vi "ProducerConsumerDataVoorbeeld.vi"() -> ()   [LabVIEW 2019]
doc: "Use this template to build a producer/consumer design pattern. Use this template when you need to execute a process, such as data analysis, when a data source, such as a triggered acquisition, produces data at an uneven rate and you need to execute the process when the data becomes available."
panel:
  in  "stop":bool
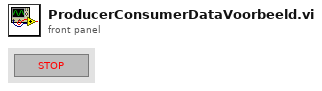
[diagram p1: front panel]
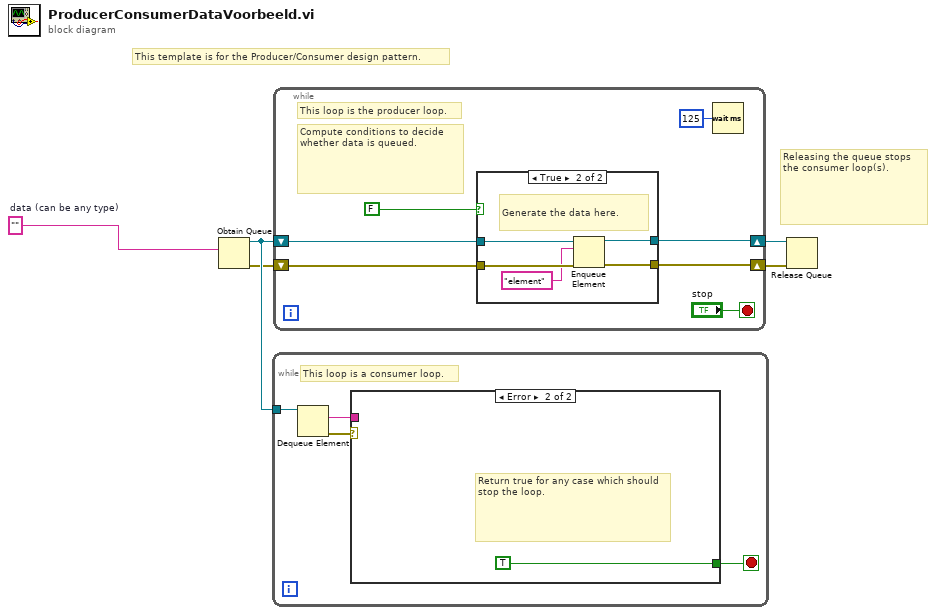
[diagram p0: block diagram]
diagram:
  w1 = ""  # data (can be any type)
  # "Releasing the queue stops the consumer loop(s)."
  # "This template is for the Producer/Consumer design pattern."
  n1 = Obtain Queue(element data type=w1) -> (queue out=w5:refnum<queue>, error out=w4:errorcluster)  [unwired: 4 in, 1 out]
  n2 = while {
    tunnel: w5 -> [w9]
    stop <- w6 stop-if-true
    # "This loop is a consumer loop."
    n3 = Dequeue Element(queue=w9) -> (element=w7:string, error out=w8:errorcluster)  [unwired: 2 in, 2 out]
    n4 = case shown="Error" w8 {
      tunnel: w7 -> [_ _]
      tunnel: [_ TRUE] -> w6
      frame No Error {
        # "This is where you process the data obtained from the queue."
      }
      frame Error {
        # "Return true for any case which should stop the loop."
      }
    }
  }
  n5 = while {
    shift-right: [w13] -> w2
    shift-left: w4 -> [w14]
    shift-right: [w15] -> w3
    shift-left: w5 -> [w16]
    stop <- "stop" stop-if-true
    # "Compute conditions to decide whether data is queued."
    # "This loop is the producer loop."
    n6 = case shown="True" FALSE ("Case Constant\n(See Context Help)") {
      tunnel: w16 -> [w19 w24]
      tunnel: [w19 w23] -> w15
      tunnel: w14 -> [w18 w22]
      tunnel: [w18 w21] -> w13
      frame False {
      }
      frame True {
        # "Generate the data here."
        n7 = Enqueue Element(queue=w24, element="element", error in (no error)=w22) -> (queue out=w23:refnum<queue>, error out=w21:errorcluster)  [unwired: 1 in, 1 out]
      }
    }
    n8 = Wait (ms)(milliseconds to wait=u32 125) -> ()  [unwired: 1 out]
  }
  n9 = Release Queue(queue=w3, error in (no error)=w2) -> ()  [unwired: 1 in, 3 out]
